vi "Write Channels.vi"(8 "error in (no error)":errorcluster, 10 "Channels":string[](array[string]), 11 "Cryo Cooler in":refnum<class "Cryo Cooler.lvclass">) -> (0 "error out":errorcluster, 3 "Cryo Cooler out":refnum<class "Cryo Cooler.lvclass">)   [LabVIEW 2024, in "Cryo Cooler.lvclass"]
uses:
  Cryo Cooler.lvclass
  Cryo Cooler.lvclass/Cryo Cooler.ctl
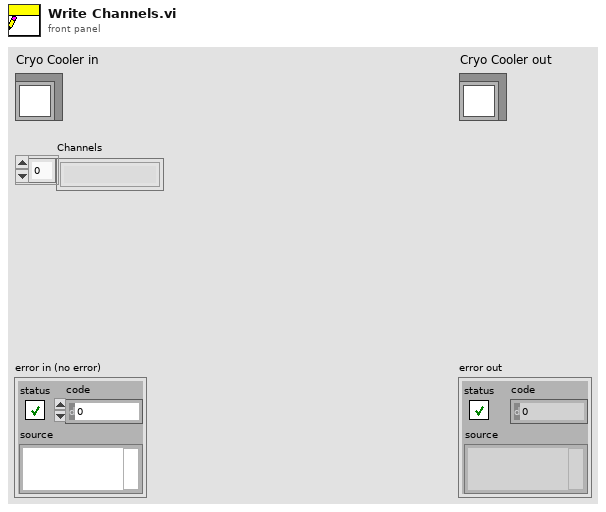
[diagram p1: front panel]
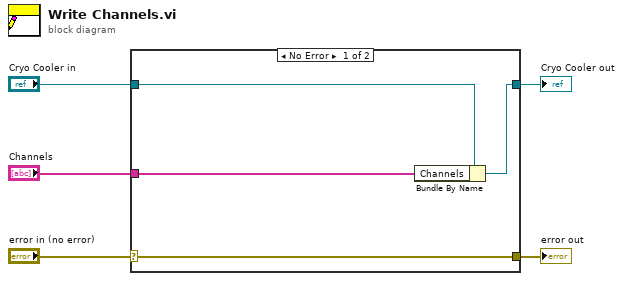
[diagram p0: block diagram]
diagram:
  n1 = case shown="No Error" "error in (no error)" {
    selector: "error in (no error)" -> [w9 w10]
    tunnel: [w9 w10] -> w4
    tunnel: [w7 w11] -> w2
    tunnel: "Cryo Cooler in" -> [w8 w11]
    tunnel: "Channels" -> [w6 _]
    frame No Error {
      n2 = Bundle By Name(cluster=w8, "Channels"=w6) -> (w7:refnum<class "Cryo Cooler.lvclass">)
    }
    frame Error {
    }
  }
  "error out" <- w4
  "Cryo Cooler out" <- w2
